vi "ProducerConsumerData 2.vi"() -> ()   [LabVIEW 2017]
doc: "Use this template to build a producer/consumer design pattern. Use this template when you need to execute a process, such as data analysis, when a data source, such as a triggered acquisition, produces data at an uneven rate and you need to execute the process when the data becomes available."
uses:
  <vilib>/Instr/_visa.llb/VISA Configure Serial Port (Instr).vi
panel:
  out "D Int out 2":i32
  in  "data":u32
  in  "idx":u16=5
  in  "DataType":enum8{"Int", " float"}(ring)=enum." float"
  in  "CommType":enum8{"Set", "Get"}(ring)
  in  "Cmd id":u16=62
  out "error out":errorcluster
  in  "error in (no error)":errorcluster
  in  "VISA resource name":refnum<visa-resource-name>="COM6"
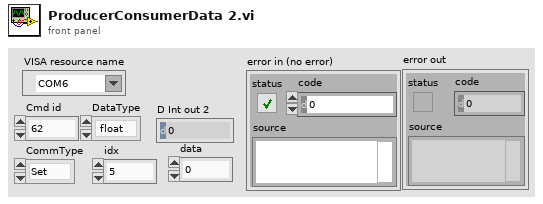
[diagram p1: front panel]
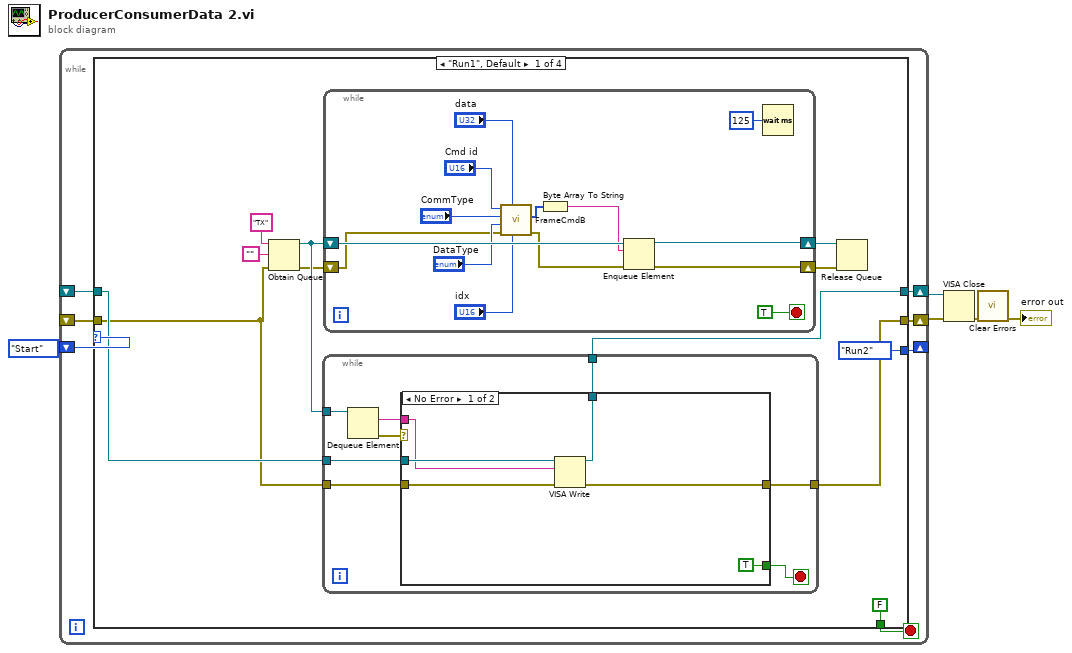
[diagram p0: block diagram]
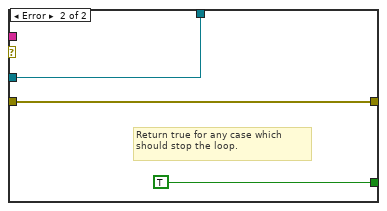
[diagram p2: hidden frame]
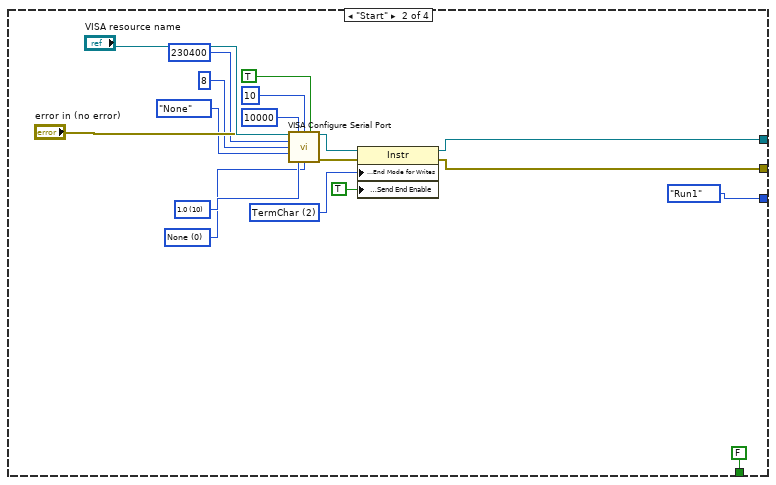
[diagram p3: hidden frame]
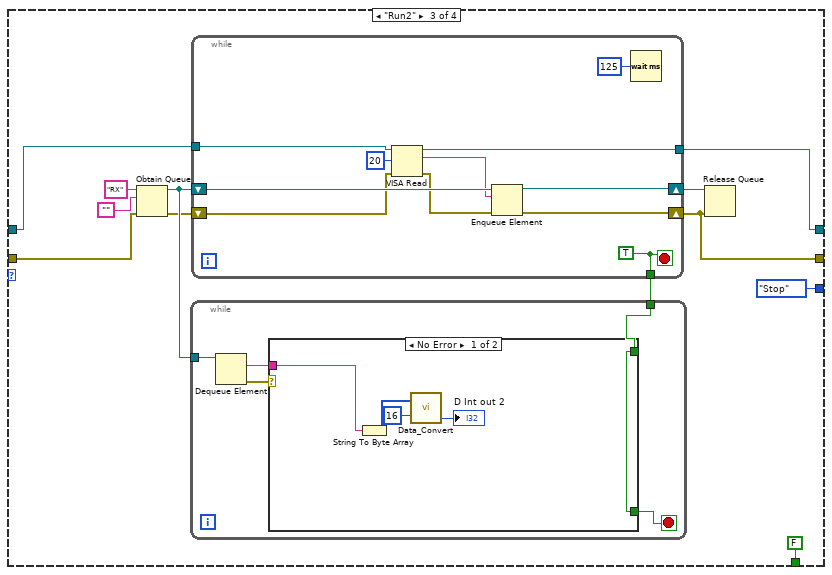
[diagram p4: hidden frame]
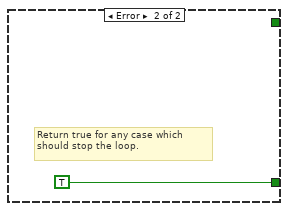
[diagram p5: hidden frame]
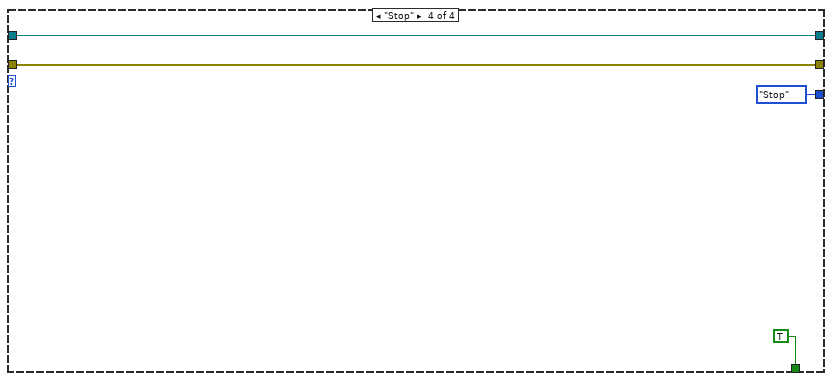
[diagram p6: hidden frame]
diagram:
  n1 = while {
    shift-right: [w11] -> w1
    shift-left: _ -> [w7]
    shift-right: [w10] -> w2
    shift-left: _ -> [w6]
    shift-right: [w9] -> _
    shift-left: enum16{"Run1", "Start", "Run2", "Stop"}."Start" -> [w12]
    stop <- w8 stop-if-true
    n2 = case shown="\"Run1\", Default" w12 {
      tunnel: [w16 w59 w76 w109] -> w11
      tunnel: [w15 w58 w74 w110] -> w10
      tunnel: [enum16{"Run1", "Start", "Run2", "Stop"}."Run2" enum16{"Run1", "Start", "Run2", "Stop"}."Run1" enum16{"Run1", "Start", "Run2", "Stop"}."Stop" enum16{"Run1", "Start", "Run2", "Stop"}."Stop"] -> w9
      tunnel: [FALSE FALSE FALSE TRUE] -> w8
      tunnel: w6 -> [w17 _ w80 w110]
      tunnel: w7 -> [w18 _ w77 w109]
      frame "Run1", Default {
        n3 = Obtain Queue(name (unnamed)="TX", element data type="", error in (no error)=w17) -> (queue out=w24:refnum<queue>, error out=w23:errorcluster)  [unwired: 2 in, 1 out]
        n4 = while {
          tunnel: w24 -> [w32]
          tunnel: w18 -> [w28]
          tunnel: w17 -> [w27]
          tunnel: [w26] -> w16
          tunnel: [w25] -> w15
          stop <- w29 stop-if-true
          n5 = Dequeue Element(queue=w32) -> (element=w30:string, error out=w31:errorcluster)  [unwired: 2 in, 2 out]
          n6 = case shown="No Error" w31 {
            tunnel: w30 -> [w36 _]
            tunnel: [TRUE TRUE] -> w29
            tunnel: w28 -> [w38 w39]
            tunnel: w27 -> [w37 w40]
            tunnel: [w35 w39] -> w26
            tunnel: [w34 w40] -> w25
            frame No Error {
              n7 = VISA Write(VISA resource name=w38, write buffer=w36, error in (no error)=w37) -> (VISA resource name out=w35:refnum<visa-resource-name>, error out=w34:errorcluster)  [unwired: 1 out]
            }
            frame Error {
              # "Return true for any case which should stop the loop."
            }
          }
        }
        n8 = while {
          shift-right: [w53] -> w21
          shift-left: w23 -> [w44]
          shift-right: [w54] -> w22
          shift-left: w24 -> [w55]
          stop <- TRUE stop-if-true
          n9 = call "FrameCmdB.vi"("idx"="idx", "data"="data", "error in"=w44, "DataType"="DataType", "CommType"="CommType", "cmd_id"="Cmd id") -> ("error out"=w43:errorcluster, "output array"=w49:u8[])  [unwired: 4 in]
          n10 = Byte Array To String(unsigned byte array=w49) -> (string=w45:string)
          n11 = Enqueue Element(queue=w55, element=w45, error in (no error)=w43) -> (queue out=w54:refnum<queue>, error out=w53:errorcluster)  [unwired: 1 in, 1 out]
          n12 = Wait (ms)(milliseconds to wait=u32 125) -> ()  [unwired: 1 out]
        }
        n13 = Release Queue(queue=w22, error in (no error)=w21) -> ()  [unwired: 1 in, 3 out]
      }
      frame "Start" {
        w61 = u16 2 items=["None", "LastBit", "TermChar", "Break"] ("Serial Settings:Serial End Mode for Writes")
        w65 = u16 0 items=["None", "XON/XOFF", "RTS/CTS", "XON/XOFF & RTS/CTS", "DTR/DSR", "XON/XOFF & DTR/DSR"] ("flow control (0:none)")
        w66 = u16 10 items=["1.0"=10, "1.5"=15, "2.0"=20] ("stop bits (10: 1 bit)")
        n14 = call-poly "VISA Configure Serial Port"("VISA resource name"="VISA resource name", "timeout (10sec)"=u32 10000, "termination char\n(0xA = '\\n' = LF)"=u8 10 ("termination char\n(0xA = '\\n' = LF)"), "Enable Termination\nChar (T)"=TRUE ("Enable Termination\nChar (T)"), "baud rate (9600)"=u32 230400, "data bits (8)"=u16 8, "parity (0:none)"=enum16{"None", "Odd", "Even", "Mark", "Space"}."None", "error in (no error)"="error in (no error)", "stop bits (10: 1 bit)"=w66, "flow control (0:none)"=w65) -> ("VISA resource name out"=w63:refnum<visa-resource-name>, "error out"=w64:errorcluster)  [unwired: 4 in]
        n15 = property class="Instr"(reference=w63, error in=w64, "Serial Settings:End Mode for Writes"=w61, "Message Based Settings:Send End Enable"=TRUE) -> (reference out=w59:refnum<visa-resource-name>, error out=w58:errorcluster)
      }
      frame "Run2" {
        n16 = Obtain Queue(name (unnamed)="RX", element data type="", error in (no error)=w80) -> (queue out=w85:refnum<queue>, error out=w84:errorcluster)  [unwired: 2 in, 1 out]
        n17 = while {
          shift-right: [w105] -> w74
          shift-left: w84 -> [w101]
          shift-right: [w106] -> w83
          shift-left: w85 -> [w107]
          tunnel: w77 -> [w99]
          tunnel: [w98] -> w76
          tunnel: [w97] -> w75
          stop <- w97 stop-if-true
          w97 = TRUE
          n18 = VISA Read(VISA resource name=w99, byte count=u32 20, error in (no error)=w101) -> (VISA resource name out=w98:refnum<visa-resource-name>, read buffer=w102:string, error out=w100:errorcluster)  [unwired: 1 out]
          n19 = Enqueue Element(queue=w107, element=w102, error in (no error)=w100) -> (queue out=w106:refnum<queue>, error out=w105:errorcluster)  [unwired: 1 in, 1 out]
          n20 = Wait (ms)(milliseconds to wait=u32 125) -> ()  [unwired: 1 out]
        }
        n21 = while {
          tunnel: w85 -> [w90]
          tunnel: w75 -> [w86]
          stop <- w87 stop-if-true
          n22 = Dequeue Element(queue=w90) -> (element=w88:string, error out=w89:errorcluster)  [unwired: 2 in, 2 out]
          n23 = case shown="No Error" w89 {
            tunnel: w88 -> [w93 _]
            tunnel: [w91 TRUE] -> w87
            tunnel: w86 -> [w91 _]
            frame No Error {
              n24 = String To Byte Array(string=w93) -> (unsigned byte array=w92:u8[])
              n25 = call "Data_Convert.vi"("Data Type"=u8 16, "Array"=w92) -> ("D Int out"=→"D Int out 2":i32)  [unwired: 2 out]
            }
            frame Error {
              # "Return true for any case which should stop the loop."
            }
          }
        }
        n26 = Release Queue(queue=w83, error in (no error)=w74) -> ()  [unwired: 1 in, 3 out]
      }
      frame "Stop" {
      }
    }
  }
  n27 = VISA Close(VISA resource name=w1, error in (no error)=w2) -> (error out=w4:errorcluster)
  n28 = call <vilib>:"Clear Errors.vi"("error in (no error)"=w4) -> ("error out"=→"error out":errorcluster)  [unwired: 5 in, 1 out]
